vi "VIDescription.vi"(11 "VersionData In":string) -> (3 "Cancelled?":bool)   [LabVIEW 2018]
doc: "*-----------------------------------------------------\n* Author: SWatts\n*\n* VI Description: Displays the VI Description\n* \n*\n* Error handling: All errors passed out\n*\n* Pre-condition: \n*\n* Post-condition: None\n*\n* Revision History:\n*\n* Rev Date Author Description \n* 01 30/04/2014 SWatts First issue\n*\n*-----------------------------------------------------"
panel:
  out "Version":string
  in  "OK":bool
  # "Input"
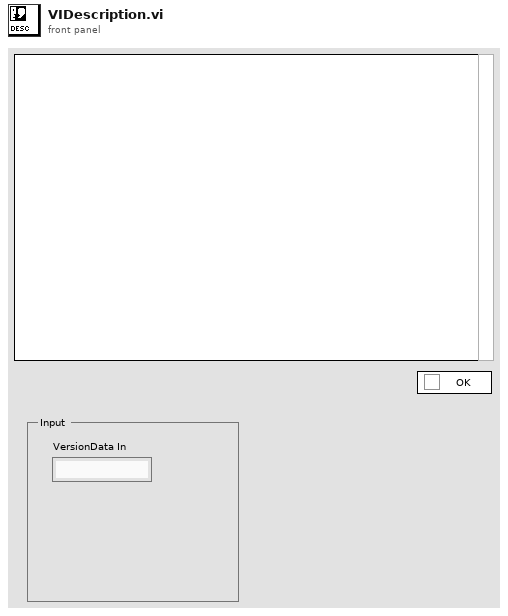
[diagram p1: front panel]
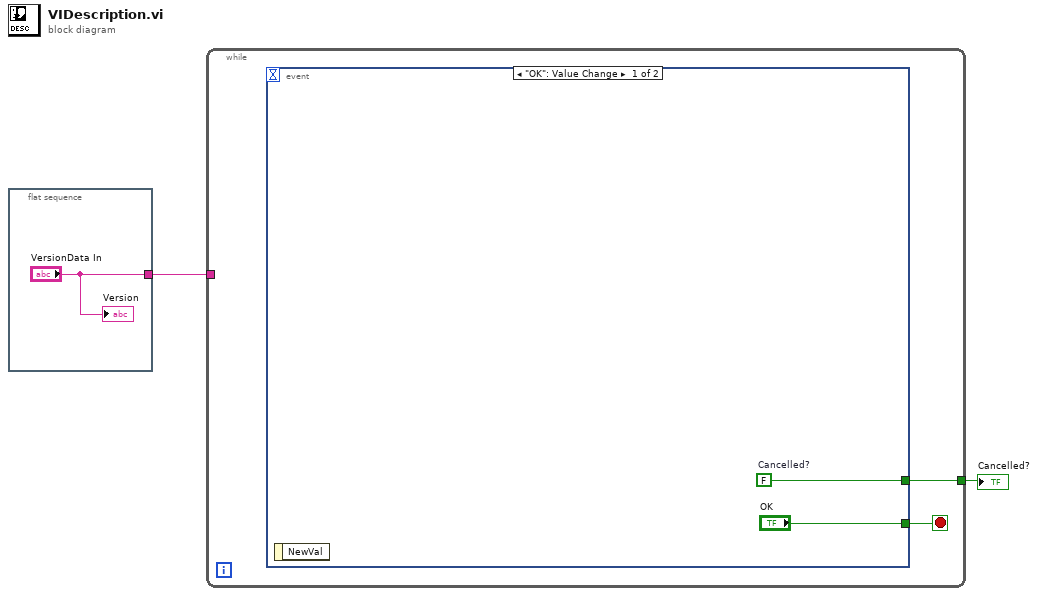
[diagram p0: block diagram]
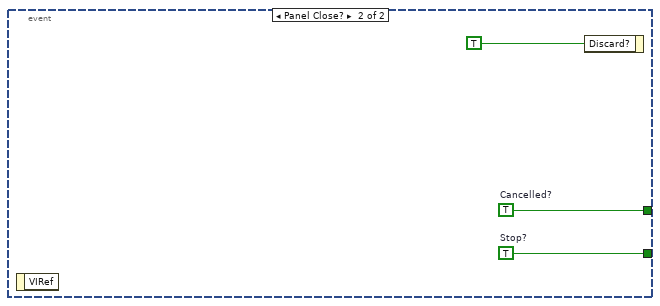
[diagram p2: hidden frame]
diagram:
  n1 = flat-sequence {
    tunnel: ["VersionData In"] -> w1
    frame #0 {
      "Version" <- "VersionData In"
    }
  }
  n2 = while {
    tunnel: [w4] -> w2
    tunnel: w1 -> [_]
    stop <- w5 stop-if-true
    n3 = event shown="[0] \"OK\": Value Change" {
      selector: _ -> [_ _]
      dyn-events: _ -> [_ _]
      timeout: _ -> [_ _]
      tunnel: ["OK" w9] -> w5
      tunnel: [w7 w8] -> w4
      event "OK": Value Change {
        w7 = FALSE  # Cancelled?
        n4 = event-data() -> ()  [unwired: 1 in, 1 out]
      }
      event Panel Close? {
        w8 = TRUE  # Cancelled?
        w9 = TRUE  # Stop?
        n5 = event-data() -> ()  [unwired: 1 in, 1 out]
        n6 = event-data("Discard?"=TRUE) -> ()  [unwired: 1 in, 1 out]
      }
    }
  }
  "Cancelled?" <- w2
